vi "Configure AC Voltage.vi"(0 "VISA resource name":refnum<visa-resource-name>, 1 "NPLC":u16(ring)=1 items=["0.00005", "1", "12", "15"], 2 "DB Reference":dbl=1.0 min=1e-07 max=1000.0, 5 "Auto Range? (T: Auto)":bool, 7 "Manual Range":dbl=10.0, 9 "Aperture Seconds":dbl, 11 "error in (no error)":errorcluster, 12 "Bandwidth (30)":u16(ring) items=["3", "30", "300"], 13 "Unit":u16(ring) items=["Volt", "DB"]) -> (4 "VISA resource name out":refnum<visa-resource-name>, 15 "error out":errorcluster)   [LabVIEW 2016, in "Keithley DMM7510.lvlib"]
doc: "This VI configures the AC Voltage measurement and the related parameters."
uses:
  Keithley DMM7510.lvlib
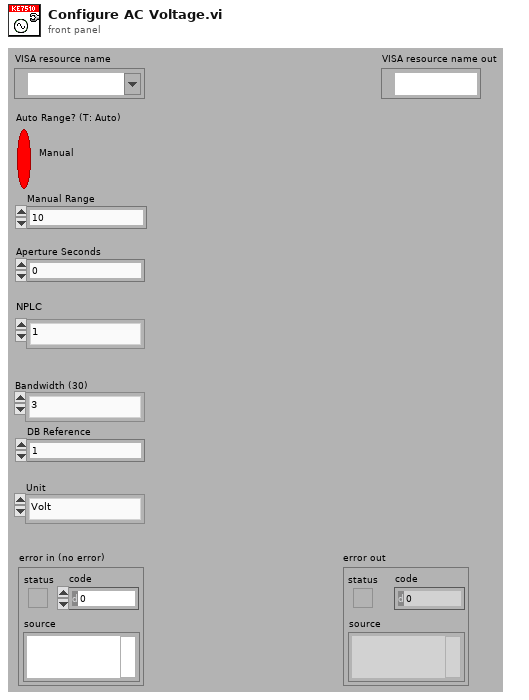
[diagram p1: front panel]
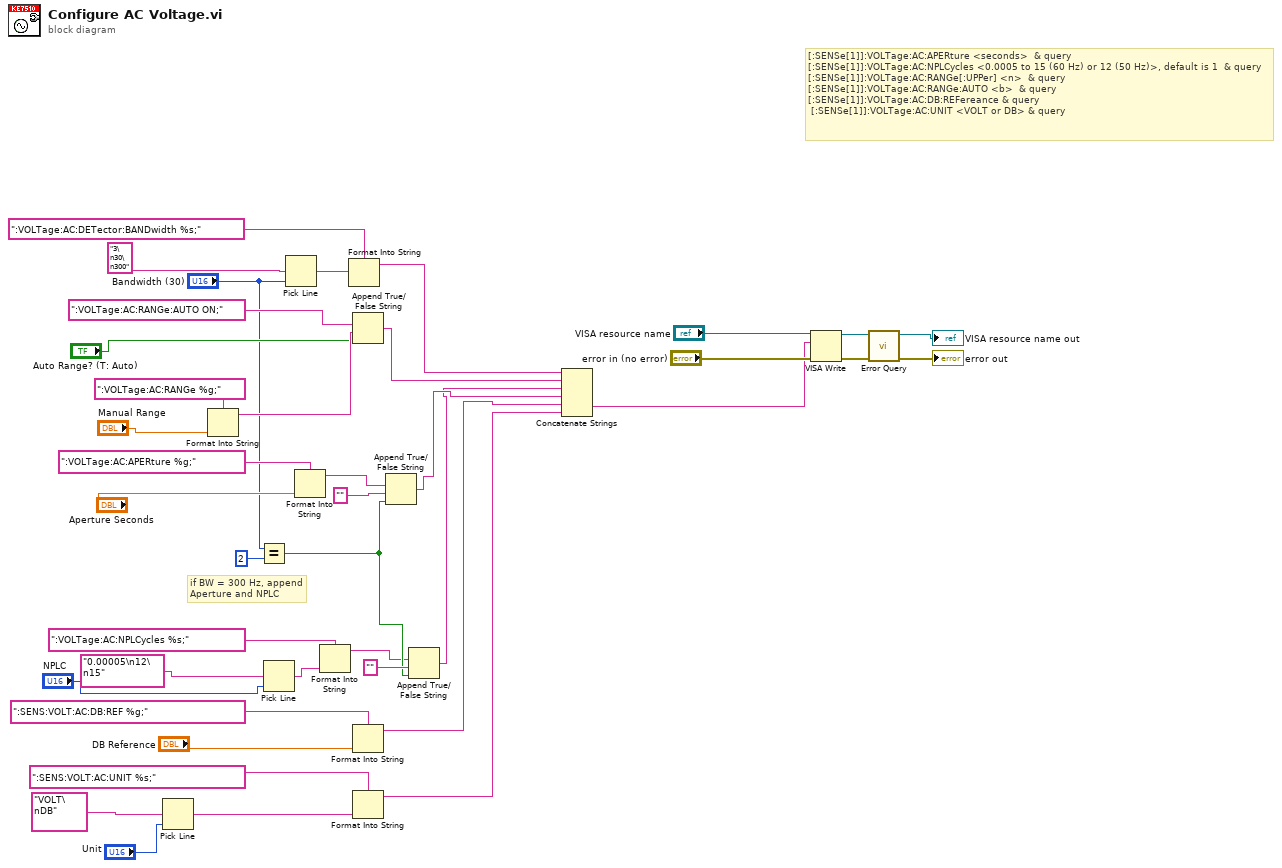
[diagram p0: block diagram]
diagram:
  # "if BW = 300 Hz, append\nAperture and NPLC"
  # "[:SENSe[1]]:VOLTage:AC:APERture <seconds>  & query\n[:SENSe[1]]:VOLTage:AC:NPLCycles <0.0005 to 15 (60 Hz) or 12 (50 Hz)>, default is 1  & query\n[:SENSe[1]]:VOLTage:AC:RANGe[:UPPer] <n>  & query\n[:SENSe[1]]:VOLTage:AC:RANGe:AUTO <b>  & query\n[:SENSe[1]]:VOLTage:AC:DB:REFereance & query\n [:SENSe[1]]:VOLTage:AC:UNIT <VOLT or DB> & query"
  n1 = Pick Line(multi-line string="VOLT\nDB", line index="Unit") -> (output string=w26:string)  [unwired: 1 in]
  n2 = Format Into String(format string=":VOLTage:AC:RANGe %g;", "Manual Range") -> (resulting string=w35:string)  [unwired: 2 in, 1 out]
  n3 = Equal?(x="Bandwidth (30)", y=u16 2) -> (x = y?=w3:bool)
  n4 = Pick Line(multi-line string="0.00005\n12\n15", line index="NPLC") -> (output string=w15:string)  [unwired: 1 in]
  n5 = Pick Line(multi-line string="3\n30\n300", line index="Bandwidth (30)") -> (output string=w18:string)  [unwired: 1 in]
  n6 = Format Into String(format string=":VOLTage:AC:APERture %g;", "Aperture Seconds") -> (resulting string=w9:string)  [unwired: 2 in, 1 out]
  n7 = Format Into String(format string=":VOLTage:AC:NPLCycles %s;", w15) -> (resulting string=w1:string)  [unwired: 2 in, 1 out]
  n8 = Format Into String(format string=":VOLTage:AC:DETector:BANDwidth %s;", w18) -> (resulting string=w10:string)  [unwired: 2 in, 1 out]
  n9 = Append True/False String(1:"Auto Range? (T: Auto)", 2:w35, 3:":VOLTage:AC:RANGe:AUTO ON;") -> (0:w32:string)  [unwired: 1 in]
  n10 = Format Into String(format string=":SENS:VOLT:AC:DB:REF %g;", "DB Reference") -> (resulting string=w24:string)  [unwired: 2 in, 1 out]
  n11 = Format Into String(format string=":SENS:VOLT:AC:UNIT %s;", w26) -> (resulting string=w23:string)  [unwired: 2 in, 1 out]
  n12 = Append True/False String(1:w3, 2:"" ("false string"), 3:w9) -> (0:w8:string)  [unwired: 1 in]
  n13 = Append True/False String(1:w3, 2:"" ("false string"), 3:w1) -> (0:w2:string)  [unwired: 1 in]
  n14 = Concatenate Strings(w10, w32, w2, w8, w24, w23) -> (w31:string)
  n15 = VISA Write(VISA resource name="VISA resource name", write buffer=w31, error in (no error)="error in (no error)") -> (VISA resource name out=w22:refnum<visa-resource-name>, error out=w21:errorcluster)  [unwired: 1 out]
  n16 = call "Error Query.vi"("error in (no error)"=w21, "VISA resource name"=w22) -> ("error out"=→"error out":errorcluster, "VISA resource name out"=→"VISA resource name out":refnum<visa-resource-name>)  [unwired: 6 in, 2 out]
